vi "Kursovaya 2.vi"() -> ()   [LabVIEW 2013]
uses:
  <instrlib>/Agilent 86100 Series/Agilent 86100 Series.lvlib
panel:
  out "VISA resource name out":refnum<visa-resource-name>
  out "error out":errorcluster
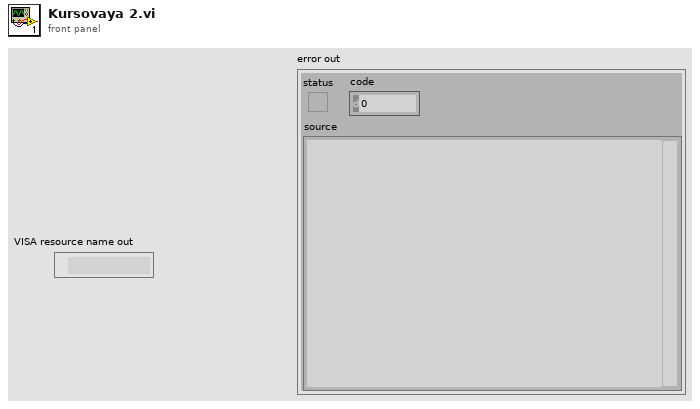
[diagram p1: front panel]
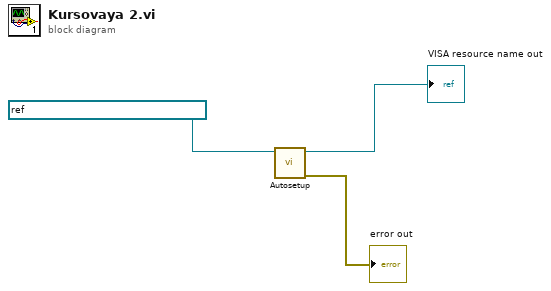
[diagram p0: block diagram]
diagram:
  n1 = call <instrlib>:"Autosetup.vi"("VISA resource name"=refnum<visa-resource-name> "TCPIP0::192.168.1.2::inst0::INSTR") -> ("error out"=→"error out":errorcluster, "VISA resource name out"=→"VISA resource name out":refnum<visa-resource-name>)  [unwired: 9 in]
